vi "HRTF-Configure Hardware (TDT).vi"(0 "Params":T2={"Fs (Hz)"=0.0, "atten (dB)"=0.0, "Waveform"=enum."Chirp", "Freq Res (Hz)"=0.0, "Order"=0, "Averages"=0, "seed"=-1, "Window"={"Type"=enum."None", "Length (ms)"=0.0, "Center (ms)"=0.0}}, 5 "State":T1, 11 "error in (no error)":errorcluster) -> (4 "Stimulus":dbl[](array[numeric]), 6 "Sample Rate (Hz)":dbl, 8 "pts/rep":i32, 10 "reps/frame":i32, 15 "error out":errorcluster)   [LabVIEW 2015]
uses:
  Typedefs/HRTF-Parameters.ctl
  Typedefs/HRTF-Waveform.ctl
  Typedefs/HRTF-Window.ctl
  Typedefs/HRTF-Window Type.ctl
  Typedefs/HRTF-State.ctl
  PXI DAQ VIs/TDT VIs/TDT-Signal Bank Action.ctl
  Typedefs/HRTF-Hardware Config (TDT).ctl
  PXI DAQ VIs/TDT VIs/Typedefs/TDT-Output source.ctl
  PXI DAQ VIs/TDT VIs/Typedefs/TDT-Device ID.ctl
  Utility VIs/Math VIs/dB to Linear (scalar).vi
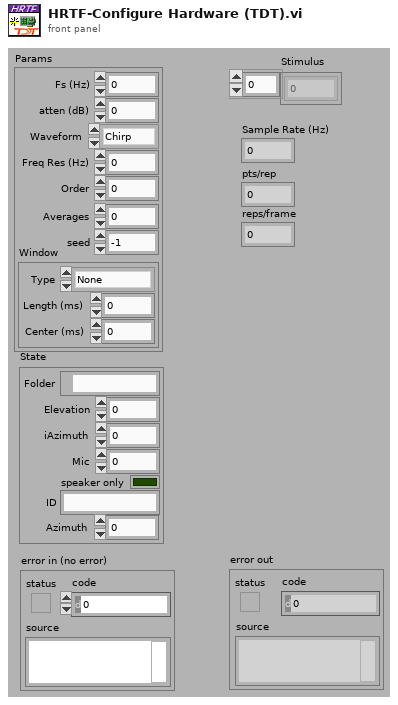
[diagram p1: front panel]
types:
  T1 = typedef "HRTF-State.ctl" = cluster{"Folder":path, "Elevation":dbl, "iAzimuth":i32, "Mic":i32, "speaker only":bool, "ID":string, "Azimuth":dbl}
  T2 = typedef "HRTF-Parameters.ctl" = cluster{"Fs (Hz)":dbl, "atten (dB)":dbl, "Waveform":T3, "Freq Res (Hz)":dbl, "Order":i32, "Averages":i32, "seed":i64, "Window":T4}
  T3 = typedef "HRTF-Waveform.ctl" = enum16{"Chirp", "MLS"}
  T4 = typedef "HRTF-Window.ctl" = cluster{"Type":T5, "Length (ms)":dbl, "Center (ms)":dbl}
  T5 = typedef "HRTF-Window Type.ctl" = enum16{"None", "Rectangle", "Hanning"}
  T6 = typedef "HRTF-Hardware Config (TDT).ctl" = cluster{"Output":T7, "Speaker":cluster{"Channel":i32, "Primary mux":i32, "Secondary mux":i32}, "Right mic":i32, "Left mic":i32}
  T7 = typedef "TDT-Output source.ctl" = cluster{"Device":T8, "Num":i32}
  T8 = typedef "TDT-Device ID.ctl" = enum16{"None", "PA5", "RP2", "RL2", "RA16", "RV8", "RX5", "RX6", "RX7", "RX8", "RZ2", "RZ5", "RZ6"}
  T9 = typedef "TDT-Signal Bank Action.ctl" = enum16{"Init", "Write", "Read", "Rewrite", "Reset", "Recycle", "Ramp up", "Ramp down", "Zero"}
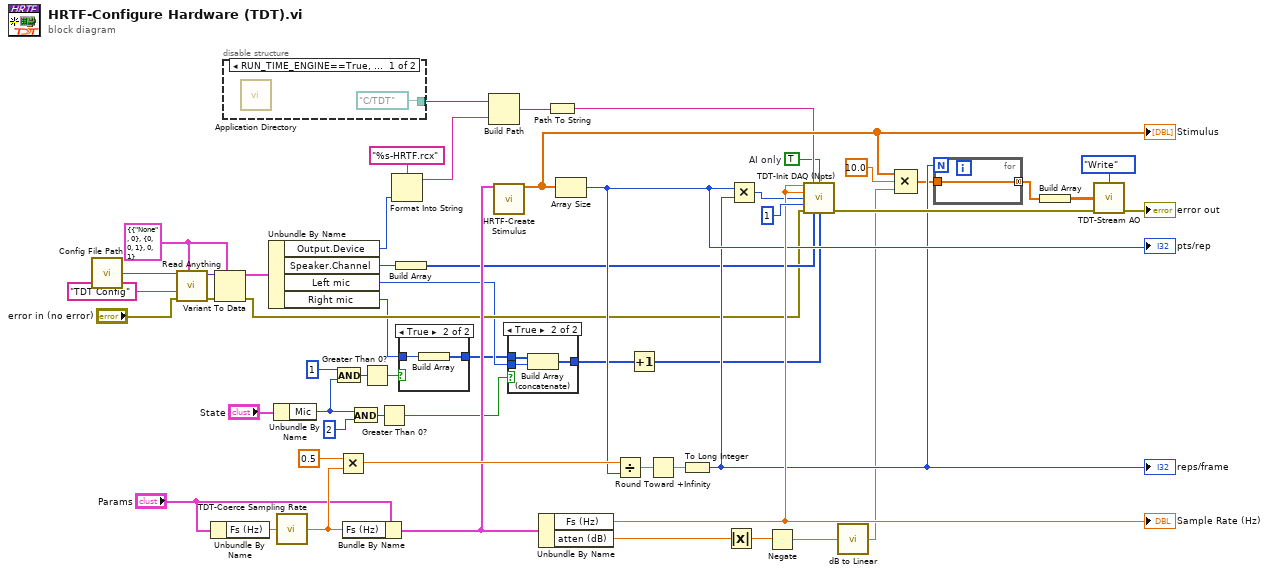
[diagram p0: block diagram]
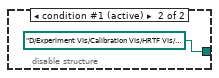
[diagram p4: hidden frame]
diagram:
  w2 = TRUE  # AI only
  w27 = T6 {"Output"={"Device"=enum."None", "Num"=0}, "Speaker"={"Channel"=0, "Primary mux"=0, "Secondary mux"=1}, "Right mic"=0, "Left mic"=1} ("TDT")
  n1 = call "Config File Path.vi"() -> ("Default config file name"=w32:path)  [unwired: 1 in]
  n2 = call "Read Anything.vi"("Type of Anything"=w27, "Error In"="error in (no error)", "Section Name (Name of \"Type of Anything\")"="TDT Config" ("Section Name (Name of \"Type of Anything\")"), "Path (dialog)"=w32) -> ("Error Out"=w35:errorcluster, "Anything"=w34:variant)  [unwired: 5 in, 1 out]
  n3 = Unbundle By Name("Params") -> ("Fs (Hz)"=w55:dbl)
  n4 = Variant To Data(error in=w35, type=w27, Variant=w34) -> (data=w28:T6, error out=w22:errorcluster)
  n5 = disable-structure shown="RUN_TIME_ENGINE==True, Default" {
    disable-tunnel: [path "C:/TDT" path "D:/Experiment VIs/Calibration VIs/HRTF VIs/rpfiles"] -> w24
    frame condition #0 {
      n6 = call <vilib>:"Application Directory.vi"() -> ()  [unwired: 1 out]
    }
    frame condition #1 (active) {
    }
  }
  n7 = Unbundle By Name(w28) -> ("Output.Device"=w20:T8, "Speaker.Channel"=w26:i32, "Left mic"=w5:i32, "Right mic"=w12:i32)
  n8 = Unbundle By Name("State") -> ("Mic"=w8:i32)
  n9 = call "TDT-Coerce Sampling Rate.vi"("Fs (Hz)"=w55) -> ("Coerced"=w45:dbl)
  n10 = And(x=1, y=w8) -> (x .and. y?=w11:i32)
  n11 = Multiply(x=0.5, y=w45) -> (x*y=w43:dbl)
  n12 = Bundle By Name(cluster="Params", "Fs (Hz)"=w45) -> (w30:T2)
  n13 = And(x=w8, y=2) -> (x .and. y?=w9:i32)
  n14 = Greater Than 0?(x=w11) -> (x > 0?=w10:bool)
  n15 = Greater Than 0?(x=w9) -> (x > 0?=w6:bool)
  n16 = Format Into String(format string="%s-HRTF.rcx", w20) -> (resulting string=w19:string)  [unwired: 2 in, 1 out]
  n17 = Build Array(w26) -> (w25:i32[])
  n18 = case shown="True" w10 {
    tunnel: w12 -> [_ w59]
    tunnel: [_ w58] -> w4
    frame False {
    }
    frame True {
      n19 = Build Array(w59) -> (w58:i32[])
    }
  }
  n20 = Build Path(base path=w24, name or relative path=w19) -> (appended path=w18:path)
  n21 = call "HRTF-Create Stimulus.vi"("Params"=w30) -> ("Stimulus"=w29:dbl[])  [unwired: 9 in, 5 out]
  "Stimulus" <- w29
  n22 = case shown="True" w6 {
    tunnel: w5 -> [_ w61]
    tunnel: [w60 w63] -> w3
    tunnel: w4 -> [w60 w62]
    frame False {
    }
    frame True {
      n23 = Build Array (concatenate)(w62, w61) -> (w63:i32[])
    }
  }
  n24 = Unbundle By Name(w30) -> ("Fs (Hz)"=w53:dbl, "atten (dB)"=w52:dbl)
  "Sample Rate (Hz)" <- w53
  n25 = Path To String(path=w18) -> (string=w17:string)
  n26 = Array Size(array=w29) -> (size(s)=w39:i32)
  "pts/rep" <- w39
  n27 = Divide(x=w43, y=w39) -> (x/y=w42:dbl)
  n28 = Increment(x=w3) -> (x+1=w1:i32[])
  n29 = Round Toward +Infinity(x=w42) -> (ceil(x): smallest int >= x=w41:dbl)
  n30 = To Long Integer(number=w41) -> (32bit integer=w38:i32)
  "reps/frame" <- w38
  n31 = Absolute Value(x=w52) -> (abs(x)=w50:dbl)
  n32 = Multiply(x=w39, y=w38) -> (x*y=w40:i32)
  n33 = Negate(x=w50) -> (-x=w51:dbl)
  n34 = call "TDT-Init DAQ (Npts).vi"("AO Fs (Hz)"=w53, "Circuit"=w17, "AI only"=w2, "AI Fs (Hz)"=w53, "Num AO Pts"=w40, "Num AO Buffers"=1, "error in (no error)"=w22, "AO Channels"=w25, "AI Channels"=w1) -> ("error out"=w48:errorcluster)  [unwired: 2 in, 4 out]
  n35 = call-poly "dB to Linear.vi"("dB"=w51) -> ("linear"=w14:dbl)
  n36 = Compound Arithmetic op=MULTIPLY(w29, 10.0 ("value"), w14) -> (w37:dbl[])
  n37 = for {
    N: w38 -> [_]
    tunnel: w37 -> [w64]
    tunnel: [w64] -> w36 mode=concatenating
  }
  n38 = Build Array(w36) -> (w46:dbl[][])
  n39 = call "TDT-Stream AO.vi"("Action"=TDT-Signal_Bank_Action."Write", "Output array"=w46, "error in (no error)"=w48) -> ("error out"=→"error out":errorcluster)  [unwired: 12 in]
